vi "Scan.vi"(0 "DMM ref":refnum<visa-resource-name>, 1 "output cluster":cluster{"Timeout":i32, "Channel number":i32}, 2 "P_current_count":i32, 3 "N_current_count":i32, 5 "DMM error":errorcluster, 7 "Current Sense \nResitance Array":dbl[](array[numeric])=[1.0032214, 1.00250644, 1.00234822, 1.0040944, 1.0017711, 1.00229431, 1.00344206, 1.00482066, 1.00381056, 1.00290978, 1.00333016, 1.00367587], 9 "ESP32 ref":refnum<visa-resource-name>, 11 "ESP32 error":errorcluster, 12 "current_mode":u8[](array[numeric])=[0, 0, 0, 0, 0, 0, 0, 0, 0, 0, 0]) -> (4 "DMM ref":refnum<visa-resource-name>, 6 "DMM error":errorcluster, 8 "Measurements":dbl[](array[numeric]), 10 "ESP32 ref":refnum<visa-resource-name>, 13 "Timout?":bool, 14 "Time out count":i32, 15 "ESP32 error":errorcluster)   [LabVIEW 2023]
uses:
  <instrlib>/Agilent 3446X Series/Agilent 3446X Series.lvlib
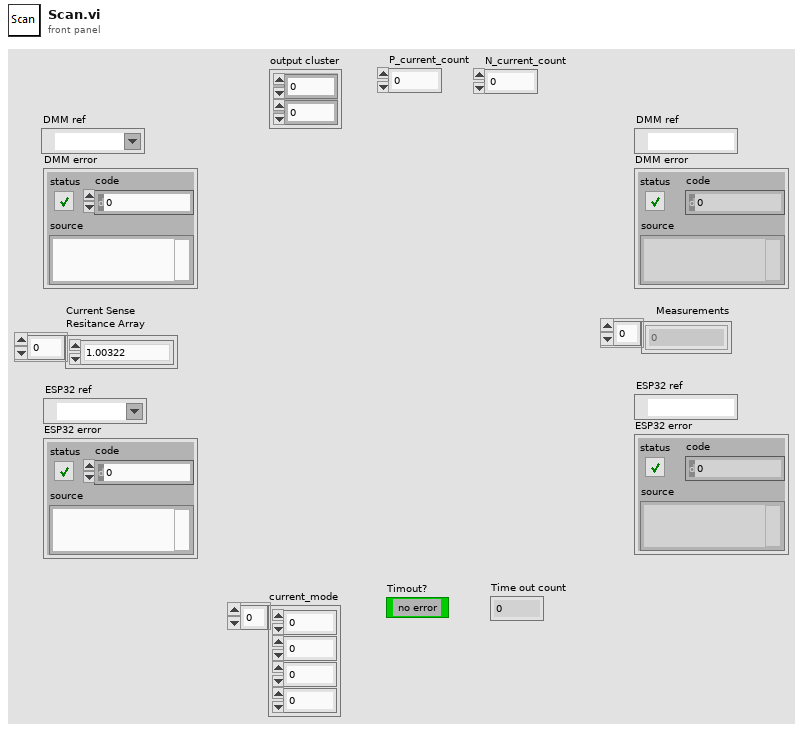
[diagram p1: front panel]
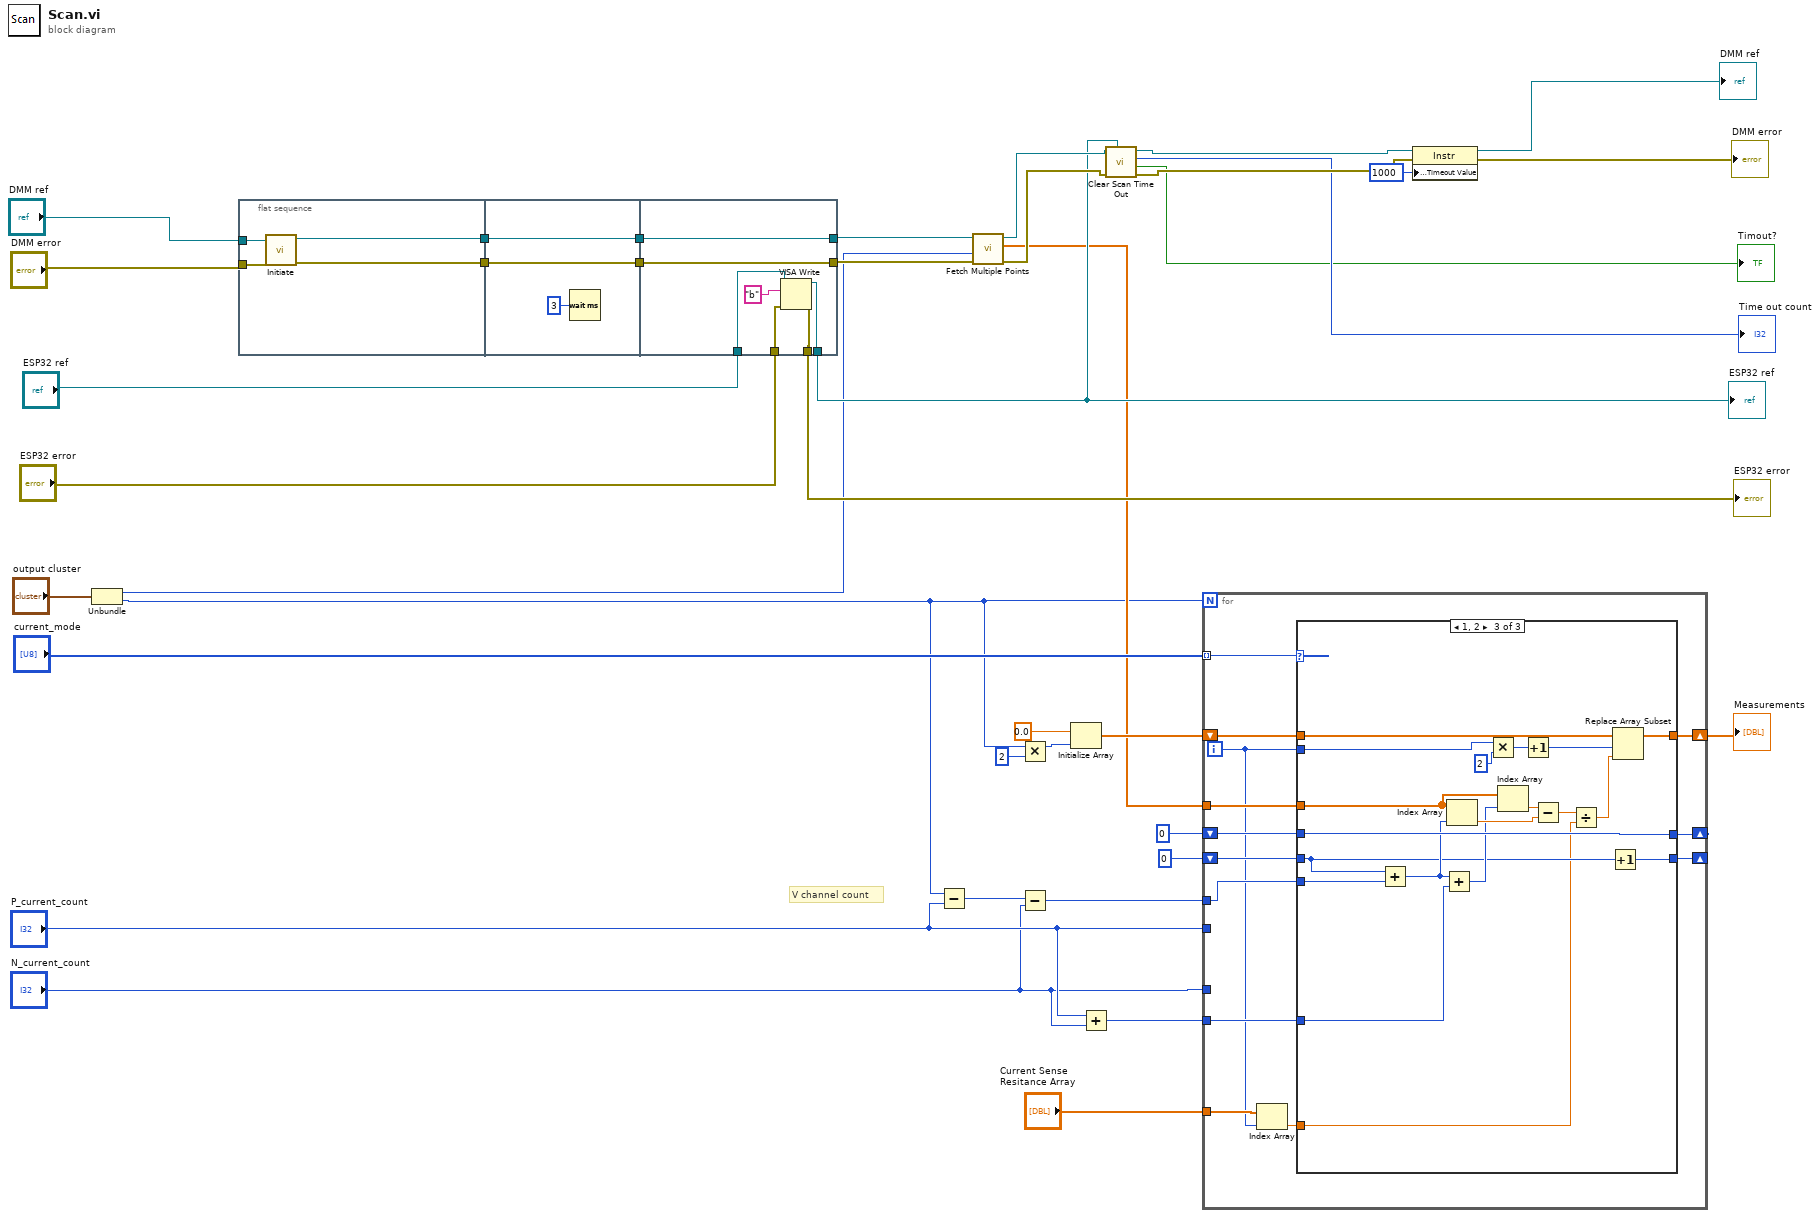
[diagram p0: block diagram]
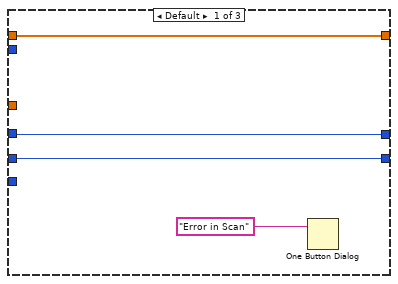
[diagram p2: hidden frame]
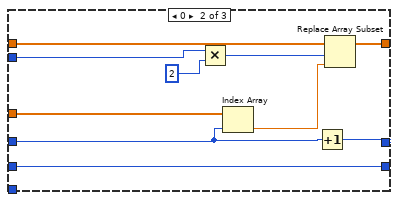
[diagram p3: hidden frame]
diagram:
  # "V channel count"
  n1 = Unbundle("output cluster") -> ("Timeout"=w1:i32, "Channel number"=w2:i32)
  n2 = flat-sequence {
    tunnel: [w43] -> w39
    tunnel: [w42] -> w38
    tunnel: "DMM ref" -> [w41]
    tunnel: "DMM error" -> [w40]
    tunnel: w39 -> [w46]
    tunnel: [w46] -> w37
    tunnel: w38 -> [w45]
    tunnel: [w45] -> w36
    tunnel: w37 -> [w53]
    tunnel: w36 -> [w52]
    tunnel: "ESP32 ref" -> [w51]
    tunnel: "ESP32 error" -> [w50]
    tunnel: [w49] -> w21
    tunnel: [w48] -> w22
    tunnel: [w53] -> w35
    tunnel: [w52] -> w34
    frame #0 {
      n3 = call <instrlib>:"Initiate.vi"("error in (no error)"=w40, "VISA resource name"=w41) -> ("error out"=w43:errorcluster, "VISA resource name out"=w42:refnum<visa-resource-name>)  [unwired: 8 in]
    }
    frame #1 {
      n4 = Wait (ms)(milliseconds to wait=u32 3) -> ()  [unwired: 1 out]
    }
    frame #2 {
      n5 = VISA Write(VISA resource name=w51, write buffer="b" ("data in"), error in (no error)=w50) -> (VISA resource name out=w49:refnum<visa-resource-name>, error out=w48:errorcluster)  [unwired: 1 out]
    }
  }
  n6 = Subtract(x=w2, y="P_current_count") -> (x-y=w12:i32)
  n7 = call <instrlib>:"Fetch Multiple Points.vi"("error in (no error)"=w35, "Timeout (10000 ms)"=w1, "VISA resource name"=w34) -> ("error out"=w30:errorcluster, "Measurements"=w13:dbl[], "VISA resource name out"=w31:refnum<visa-resource-name>)  [unwired: 1 in, 5 out]
  n8 = Multiply(x=w2, y=2) -> (x*y=w17:i32)
  n9 = Subtract(x=w12, y="N_current_count") -> (x-y=w11:i32)
  n10 = Initialize Array(0.0 ("Measurement"), w17) -> (w15:dbl[])
  n11 = Add(x="P_current_count", y="N_current_count") -> (x+y=w6:i32)
  n12 = call "Clear Scan Time Out.vi"("ESP32 ref"=w21, "error in (no error)"=w30, "VISA Refnum in"=w31) -> ("error out"=w28:errorcluster, "error?"=→"Timout?":bool, "Time out count"=→"Time out count":i32, "VISA Refnum out"=w29:refnum<visa-resource-name>)  [unwired: 4 in, 1 out]
  n13 = for {
    N: w2 -> [_]
    shift-right: [w61] -> w5
    shift-left: w15 -> [w62]
    tunnel: "current_mode" -> [w66] mode=indexing
    tunnel: w13 -> [w65]
    tunnel: "P_current_count" -> [_]
    tunnel: "N_current_count" -> [_]
    tunnel: w11 -> [w58]
    shift-right: [w63] -> _
    shift-left: 0 ("index") -> [w64]
    shift-right: [w59] -> _
    shift-left: 0 ("index") -> [w60]
    tunnel: w6 -> [w57]
    tunnel: "Current Sense \nResitance Array" -> [w56]
    i -> [w55]
    n14 = Index Array(array=w56, index=w55) -> (element=w54:dbl)
    n15 = case shown="1, 2" w66 {
      tunnel: w65 -> [_ w80 w92]
      tunnel: w64 -> [w70 w78 w93]
      tunnel: [w70 w77 w93] -> w63
      tunnel: w55 -> [_ w75 w98]
      tunnel: w62 -> [w69 w76 w99]
      tunnel: [w69 w73 w95] -> w61
      tunnel: w60 -> [w68 w72 w85]
      tunnel: [w68 w72 w84] -> w59
      tunnel: w58 -> [_ _ w89]
      tunnel: w57 -> [_ _ w88]
      tunnel: w54 -> [_ _ w82]
      frame Default {
        n16 = One Button Dialog(message="Error in Scan") -> ()  [unwired: 1 in, 1 out]
      }
      frame 0 {
        n17 = Multiply(x=w75, y=2 ("x")) -> (x*y=w71:i32)
        n18 = Index Array(array=w80, index=w78) -> (element=w79:dbl)
        n19 = Increment(x=w78) -> (x+1=w77:i32)
        n20 = Replace Array Subset(array=w76, new element=w79, index=w71) -> (w73:dbl[])
      }
      frame 1, 2 {
        n21 = Add(x=w85, y=w89) -> (x+y=w87:i32)
        n22 = Add(x=w87, y=w88) -> (x+y=w86:i32)
        n23 = Index Array(array=w92, index=w87) -> (element=w90:dbl)
        n24 = Multiply(x=w98, y=2 ("x")) -> (x*y=w96:i32)
        n25 = Index Array(array=w92, index=w86) -> (element=w91:dbl)
        n26 = Increment(x=w96) -> (x+1=w94:i32)
        n27 = Subtract(x=w91, y=w90) -> (x-y=w83:dbl)
        n28 = Divide(x=w83, y=w82) -> (x/y=w81:dbl)
        n29 = Increment(x=w85) -> (x+1=w84:i32)
        n30 = Replace Array Subset(array=w99, new element=w81, index=w94) -> (w95:dbl[])
      }
    }
  }
  "Measurements" <- w5
  n31 = property class="Instr"(reference=w29, error in=w28, "General Settings:Timeout Value"=u32 1000) -> (reference out=→"DMM ref":refnum<visa-resource-name>, error out=→"DMM error":errorcluster)
  "ESP32 ref" <- w21
  "ESP32 error" <- w22
